vi "loadDocument.vi"(8 "error in (no error)":errorcluster, 11 "MS-Word in":refnum<class "MS-Word.lvclass">) -> (0 "error out":errorcluster, 3 "MS-Word out":refnum<class "MS-Word.lvclass">)   [LabVIEW 2017, in "LabVIEW NPOI.lvlib" / "MS-Word.lvclass"]
uses:
  MS-Word.lvclass
  MS-Word.lvclass/MS-Word.ctl
  xwpfReader/xwpfReader.lvclass
  xwpfWriter/xwpfWriter.lvclass
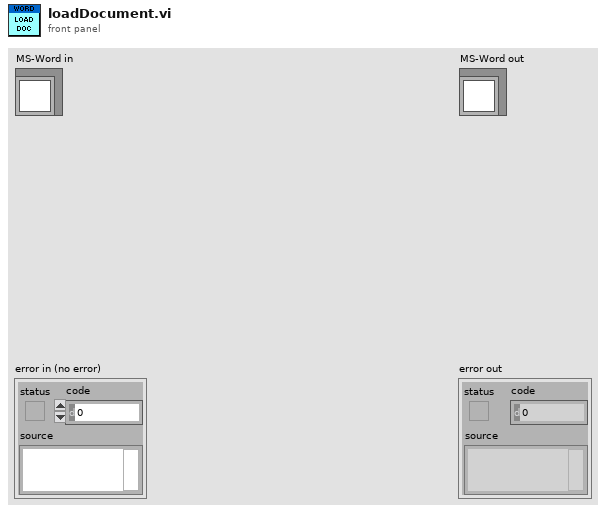
[diagram p1: front panel]
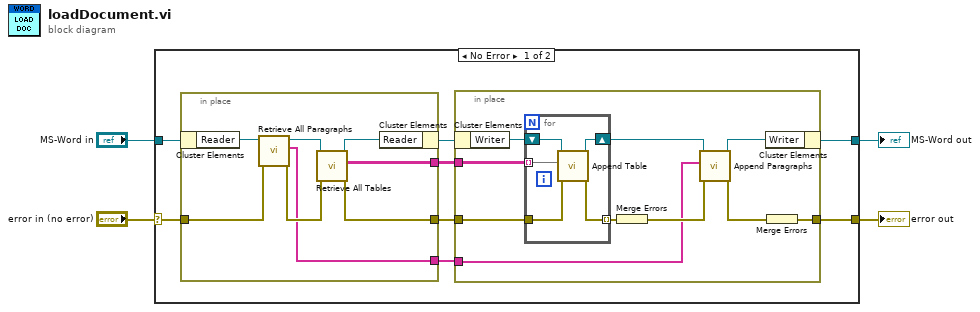
[diagram p0: block diagram]
diagram:
  n1 = case shown="No Error" "error in (no error)" {
    selector: "error in (no error)" -> [w10 w37]
    tunnel: [w5 w37] -> w3
    tunnel: [w12 w36] -> w1
    tunnel: "MS-Word in" -> [w11 w36]
    frame No Error {
      n2 = in-place {
        in-place-border: w10 -> [w32]
        in-place-border: [w30] -> w8
        in-place-border: [w29] -> w7
        in-place-border: [w28] -> w6
        n3 = in-place-cluster #1(w11) -> ("Reader"=w35:refnum<class "xwpfReader.lvclass">)
        n4 = call "Retrieve All Paragraphs.vi"("error in (no error)"=w32, "xwpfReader in"=w35) -> ("error out"=w31:errorcluster, "Paragraphs"=w28:string[], "xwpfReader out"=w34:refnum<class "xwpfReader.lvclass">)  [unwired: 7 in]
        n5 = call "Retrieve All Tables.vi"("error in (no error)"=w31, "xwpfReader in"=w34) -> ("error out"=w30:errorcluster, "Tables"=w29:string[][][], "xwpfReader out"=w33:refnum<class "xwpfReader.lvclass">)  [unwired: 7 in]
        n6 = in-place-cluster #1("Reader"=w33) -> (w9:refnum<class "MS-Word.lvclass">)
      }
      n7 = in-place {
        in-place-border: w8 -> [w20]
        in-place-border: w7 -> [w21]
        in-place-border: [w14] -> w5
        in-place-border: w6 -> [w13]
        n8 = in-place-cluster #2(w9) -> ("Writer"=w22:refnum<class "xwpfWriter.lvclass">)
        n9 = for {
          tunnel: w21 -> [w25] mode=indexing
          shift-right: [w26] -> w18
          shift-left: w22 -> [w27]
          tunnel: w20 -> [w24]
          tunnel: [w23] -> w19 mode=indexing
          n10 = call "Append Table.vi"("error in (no error)"=w24, "Table"=w25, "xwpfWriter in"=w27) -> ("error out"=w23:errorcluster, "xwpfWriter out"=w26:refnum<class "xwpfWriter.lvclass">)  [unwired: 7 in]
        }
        n11 = Merge Errors(w19) -> (w16:errorcluster)
        n12 = call "Append Paragraphs.vi"("error in (no error)"=w16, "Paragraphs"=w13, "xwpfWriter in"=w18) -> ("error out"=w15:errorcluster, "xwpfWriter out"=w17:refnum<class "xwpfWriter.lvclass">)  [unwired: 7 in]
        n13 = in-place-cluster #2("Writer"=w17) -> (w12:refnum<class "MS-Word.lvclass">)
        n14 = Merge Errors(w15) -> (w14:errorcluster)
      }
    }
    frame Error {
    }
  }
  "error out" <- w3
  "MS-Word out" <- w1
